vi "Configure Trigger (Setup & Hold Extended).vi"(0 "VISA resource name":refnum<visa-resource-name>, 1 "Data Threshold (9.91E+37 V)":dbl=9.91e+37, 5 "Channel (0: Channel 1)":i32(ring) items=["Channel 1", "Channel 2", "Channel 3", "Channel 4", "Digital Channel 0", "Digital Channel 1", "Digital Channel 2", "Digital Channel 3", "Digital Channel 4", "Digital Channel 5", "Digital Channel 6", "Digital Channel 7", "Digital Channel 8", "Digital Channel 9", "Digital Channel 10", "Digital Channel 11", "Digital Channel 12", "Digital Channel 13", "Digital Channel 14", "Digital Channel 15"], 7 "Threshold (0 V)":dbl, 9 "Clock Threshold (0 V)":dbl, 11 "error in (no error)":errorcluster) -> (4 "VISA resource name out":refnum<visa-resource-name>, 15 "error out":errorcluster)   [LabVIEW 2009, in "Tektronix DPO MSO 2000 4000 Series.lvlib"]
doc: "Configures voltage threshold, clock threshold and data voltage threshold for sethold trigger for an oscilloscope. A sethold trigger occurs when a setup or hold violation happens.\n\n<B>Note:</B>\n\n<B>Configure Trigger (Setup & Hold)</B> VI should be called before this VI."
uses:
  <instrlib>/Tektronix DPO MSO 2000 4000 Series/Tektronix DPO MSO 2000 4000 Series.lvlib
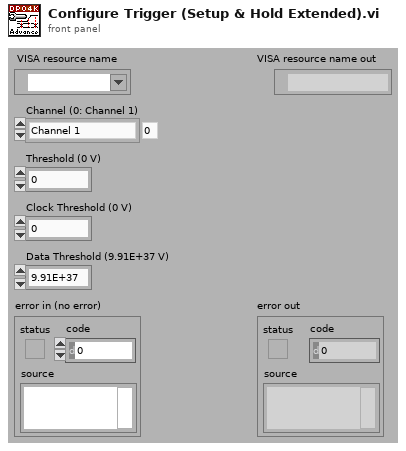
[diagram p1: front panel]
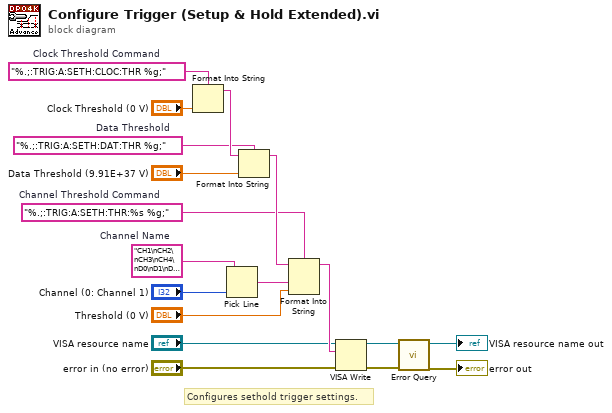
[diagram p0: block diagram]
diagram:
  w10 = "%.;:TRIG:A:SETH:THR:%s %g;"  # Channel Threshold Command
  w13 = "CH1\nCH2\nCH3\nCH4\nD0\nD1\nD2\nD3\nD4\nD5\nD6\nD7\nD8\nD9\nD10\nD11\nD12\nD13\nD14\nD15"  # Channel Name
  w15 = "%.;:TRIG:A:SETH:DAT:THR %g;"  # Data Threshold
  w18 = "%.;:TRIG:A:SETH:CLOC:THR %g;"  # Clock Threshold Command
  # "Configures sethold trigger settings."
  n1 = Format Into String(format string=w18, "Clock Threshold (0 V)") -> (resulting string=w16:string)  [unwired: 2 in, 1 out]
  n2 = Pick Line(multi-line string=w13, line index="Channel (0: Channel 1)") -> (output string=w9:string)  [unwired: 1 in]
  n3 = Format Into String(format string=w15, initial string=w16, "Data Threshold (9.91E+37 V)") -> (resulting string=w11:string)  [unwired: 1 in, 1 out]
  n4 = Format Into String(format string=w10, initial string=w11, w9, "Threshold (0 V)") -> (resulting string=w7:string)  [unwired: 1 in, 1 out]
  n5 = VISA Write(VISA resource name="VISA resource name", write buffer=w7, error in (no error)="error in (no error)") -> (VISA resource name out=w4:refnum<visa-resource-name>, error out=w3:errorcluster)  [unwired: 1 out]
  n6 = call <instrlib>:"Error Query.vi"("error in (no error)"=w3, "VISA resource name"=w4) -> ("error out"=→"error out":errorcluster, "VISA resource name out"=→"VISA resource name out":refnum<visa-resource-name>)  [unwired: 6 in, 2 out]
